vi "add delta initalize(SubVI).vi"(9 "字符串":string, 10 "model":string="Delta") -> (0 "连接的字符串":string, 3 "ok or cancel":bool=TRUE)   [LabVIEW 2019, in "Add Seq.lvlib"]
uses:
  Add Seq.lvlib
  lib/Keithley 622x/Configure/Delta PDelta DCon Modes/Typedefs/KE622x -- Delta Mode Params.ctl
  lib/Keithley 622x/Configure/Delta PDelta DCon Modes/Low Level/Typedefs/KE622x -- Delta PDelta Mode High Level.ctl
  lib/Keithley 622x/Configure/Delta PDelta DCon Modes/Low Level/Typedefs/KE622x -- Delta PDelta Mode Low Level.ctl
  lib/Keithley 622x/Configure/Delta PDelta DCon Modes/Low Level/Typedefs/KE622x -- Delta DCon Mode Delay.ctl
  lib/Keithley 622x/Configure/Delta PDelta DCon Modes/Low Level/Typedefs/KE622x -- Delta PDelta Mode Num Cycles Mode.ctl
  lib/Keithley 622x/Configure/Delta PDelta DCon Modes/Low Level/Typedefs/KE622x -- Delta PDelta Mode Num Cycles.ctl
  lib/Keithley 622x/Configure/2182 -A/Low Level/Typedefs/KE2182 -- Voltage Ranges.ctl
  lib/Keithley 622x/Configure/2182 -A/Low Level/Typedefs/KE2182 -- Filter Type.ctl
  lib/Keithley 622x/Configure/2182 -A/Low Level/Typedefs/KE2182 -- Filter Count.ctl
  lib/Keithley 622x/Configure/2182 -A/Low Level/Typedefs/KE2182 -- Filter Window.ctl
  lib/Keithley 622x/Configure/2182 -A/Low Level/Typedefs/KE2182 -- NPLCs.ctl
  SubVI.lvlib
  lib/Keithley 622x/Keithley 622x.lvlib
panel:
  out "错误输出":errorcluster
  in  "load":bool
  in  "2812 -A Params In":T6={"Auto Range?"=FALSE, "Man / Selected\nRange"=enum."10mV", "Enable Digital\nFilter?"=FALSE, "Filter Type"=enum."Moving", "Filter Count"=10, "Filter\nWindow (%)"=0.01, "Enable Analog\nFilter?"=FALSE, "NPLCs"=5} {"Filter\nWindow (%)" min=0.0 max=10.0 step=0.01 format="%.2f"; "Filter Count" min=1 max=100; "NPLCs" min=1 max=10}
  in  "Delta Mode Params In":T7={"High Level (A)"=0.001, "Low Level (A)"=-0.001, "Delay (s)"=0.02, "Num Cycles Mode"=enum."Finite Count", "Finite Count"=6, "Abort On\nCompliance?"=FALSE, "Cold Swithing\nMode Enabled?"=FALSE} {"Finite Count" min=1 max=65536; "Low Level (A)" min=-0.105 max=0.0 format="%.3p"; "High Level (A)" min=0.0 max=0.105 format="%.3p"; "Delay (s)" min=0.001 max=9999.999 format="%.3f"}
  in  "cancel":bool
  in  "ok":bool
  in  "6221 Resource":refnum<visa-resource-name>="GPIB1::10::INSTR"
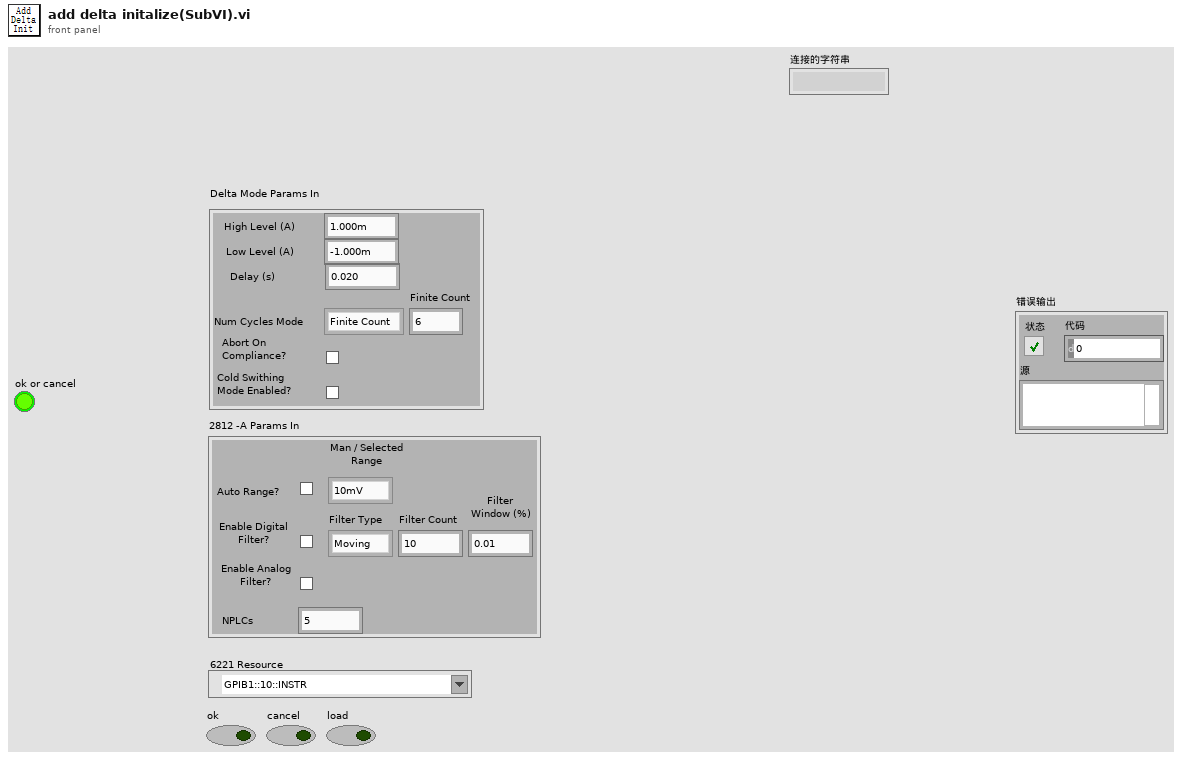
[diagram p1: front panel]
types:
  T1 = typedef "Keithley 622x.lvlib/KE2182 -- Voltage Ranges.ctl" = enum16{"10mV", "100mV", "1V", "10V", "100V"}
  T2 = typedef "Keithley 622x.lvlib/KE2182 -- Filter Type.ctl" = enum16{"Moving", "Repeat"}
  T3 = typedef "Keithley 622x.lvlib/KE2182 -- Filter Count.ctl" = u32
  T4 = typedef "Keithley 622x.lvlib/KE2182 -- Filter Window.ctl" = dbl
  T5 = typedef "Keithley 622x.lvlib/KE2182 -- NPLCs.ctl" = u32
  T6 = cluster{"Auto Range?":bool, "Man / Selected\nRange":T1, "Enable Digital\nFilter?":bool, "Filter Type":T2, "Filter Count":T3, "Filter\nWindow (%)":T4, "Enable Analog\nFilter?":bool, "NPLCs":T5}
  T7 = typedef "Keithley 622x.lvlib/KE622x -- Delta Mode Params.ctl" = cluster{"High Level (A)":T8, "Low Level (A)":T9, "Delay (s)":T10, "Num Cycles Mode":T11, "Finite Count":T12, "Abort On\nCompliance?":bool, "Cold Swithing\nMode Enabled?":bool}
  T8 = typedef "Keithley 622x.lvlib/KE622x -- Delta PDelta Mode High Level.ctl" = dbl
  T9 = typedef "Keithley 622x.lvlib/KE622x -- Delta PDelta Mode Low Level.ctl" = dbl
  T10 = typedef "Keithley 622x.lvlib/KE622x -- Delta DCon Mode Delay.ctl" = dbl
  T11 = typedef "Keithley 622x.lvlib/KE622x -- Delta PDelta Mode Num Cycles Mode.ctl" = enum16{"Finite Count", "Infinite"}
  T12 = typedef "Keithley 622x.lvlib/KE622x -- Delta PDelta Mode Num Cycles.ctl" = u32
  T13 = enum16{"open", "replace", "create", "open or create", "replace or create"}
  T14 = enum16{"open", "replace", "create", "open or create", "replace or create", "replace or create with confirmation"}
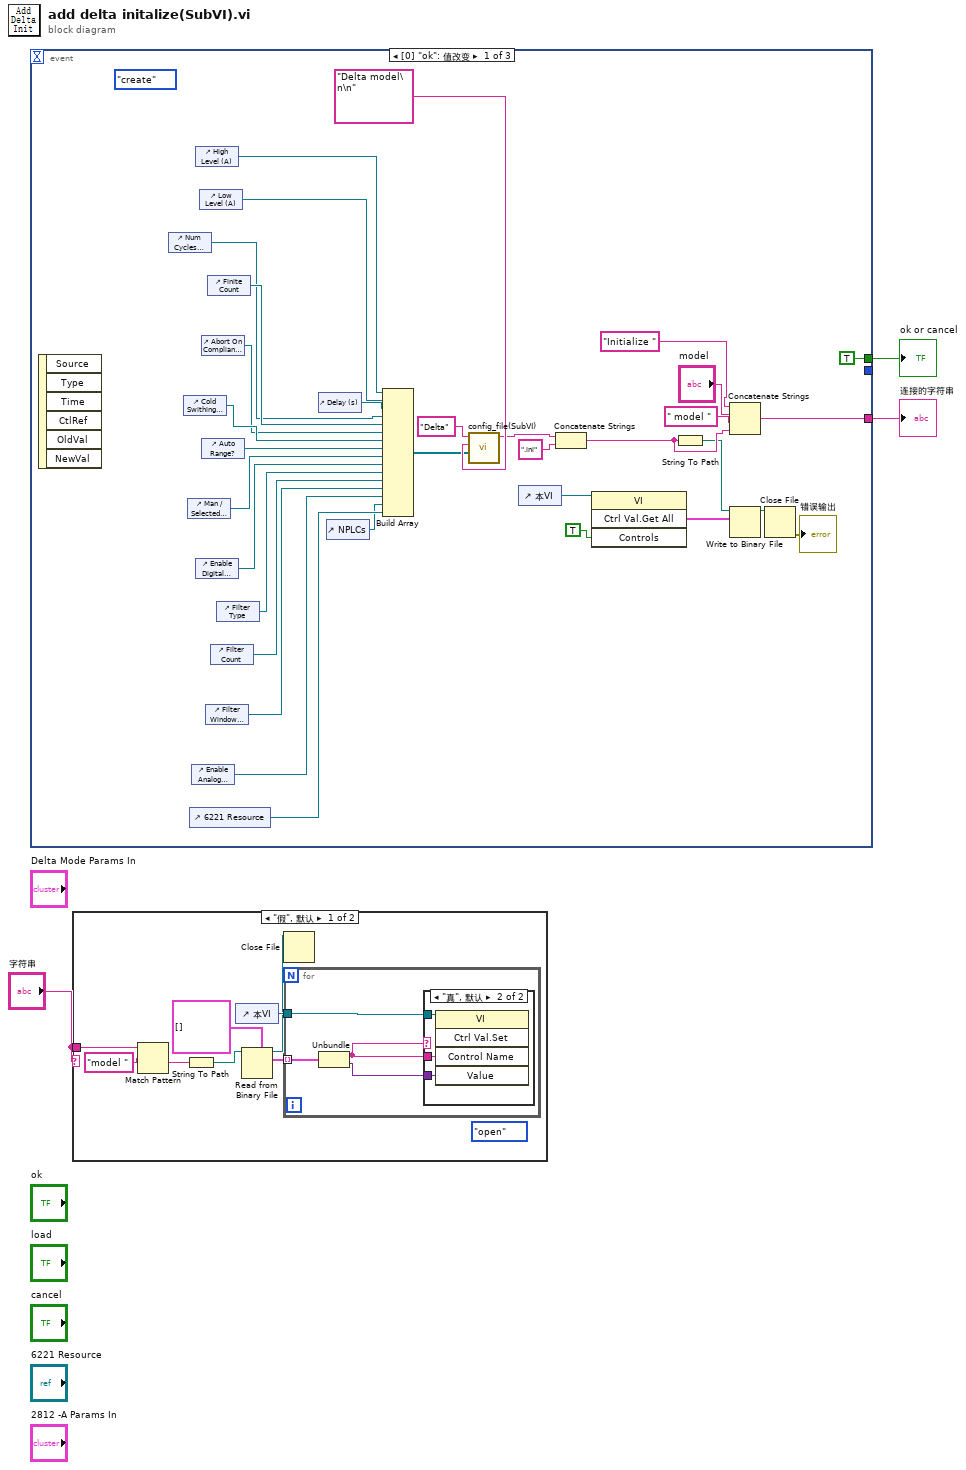
[diagram p0: block diagram]
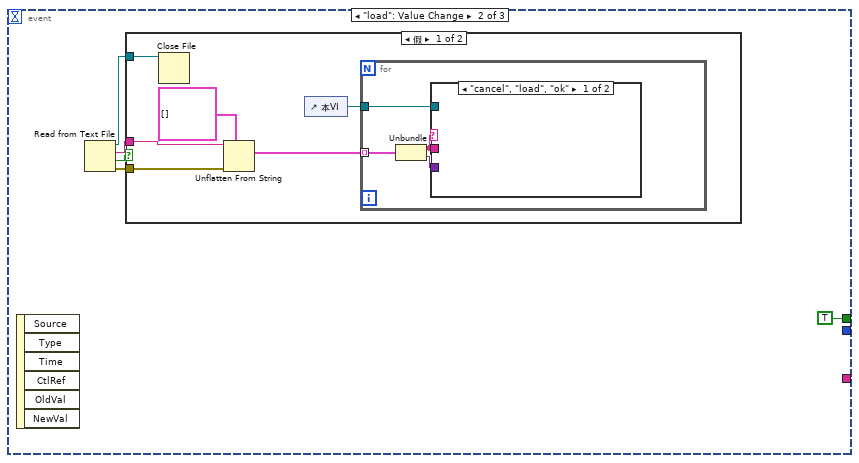
[diagram p4: hidden frame]
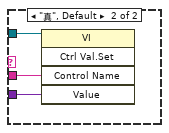
[diagram p5: hidden frame]
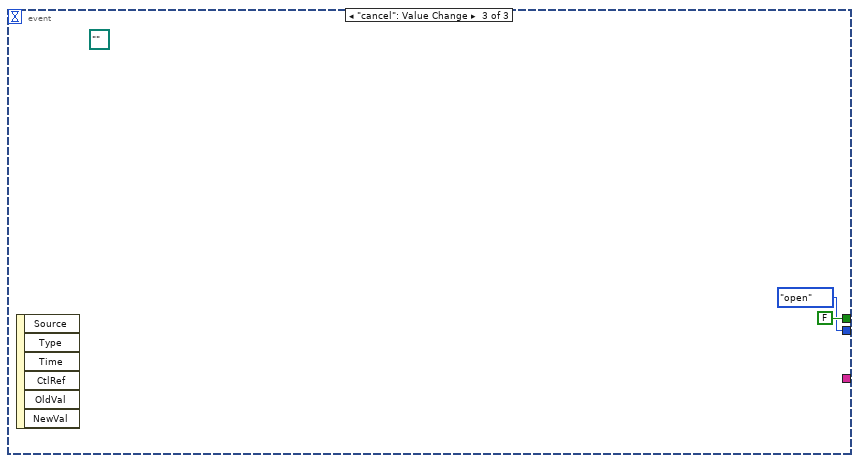
[diagram p7: hidden frame]
diagram:
  n1 = event shown="[0] \"ok\": 值改变" {
    selector: _ -> [_ _ _]
    dyn-events: _ -> [_ _ _]
    timeout: _ -> [_ _ _]
    tunnel: [_ _ T13."open" ("operation(0:open)")] -> _
    tunnel: [TRUE TRUE FALSE] -> w3
    tunnel: [w7 _ _] -> w2
    event "ok": Value Change {
      (unwired) T14."create" ("操作(0:open)")
      n2 = event-data() -> ()  [unwired: 1 in, 6 out]
      n3 = control-ref of="Num Cycles Mode"() -> (w15:refnum<vi>)
      n4 = control-ref of="Cold Swithing\nMode Enabled?"() -> (w18:refnum<vi>)
      n5 = control-ref of="Man / Selected\nRange"() -> (w20:refnum<vi>)
      n6 = control-ref of="6221 Resource"() -> (w27:refnum<vi>)
      n7 = control-ref of="Enable Analog\nFilter?"() -> (w25:refnum<vi>)
      n8 = control-ref of="High Level (A)"() -> (w12:refnum<vi>)
      n9 = control-ref of="Enable Digital\nFilter?"() -> (w21:refnum<vi>)
      n10 = control-ref of="Low Level (A)"() -> (w13:refnum<vi>)
      n11 = control-ref of="Abort On\nCompliance?"() -> (w17:refnum<vi>)
      n12 = control-ref of="Auto Range?"() -> (w19:refnum<vi>)
      n13 = control-ref of="Filter\nWindow (%)"() -> (w24:refnum<vi>)
      n14 = control-ref of="Finite Count"() -> (w16:refnum<vi>)
      n15 = control-ref of="Filter Count"() -> (w23:refnum<vi>)
      n16 = control-ref of="Filter Type"() -> (w22:refnum<vi>)
      n17 = control-ref of="Delay (s)"() -> (w14:refnum<vi>)
      n18 = control-ref of="NPLCs"() -> (w26:refnum<vi>)
      n19 = Build Array(w12, w13, w14, w15, w16, w17, w18, w19, w20, w21, w22, w23, w24, w25, w26, w27) -> (w10:refnum<vi>[])
      n20 = call "config_file(SubVI).vi"("all ref"=w10, "文件抬头"="Delta model\n\n", "文件夹名称"="Delta" ("字符串")) -> ("字符串输出"=w30:string)  [unwired: 8 in]
      n21 = control-ref of="本VI"() -> (w33:refnum<vi>)
      n22 = Concatenate Strings(w30, ".ini" ("字符串")) -> (w28:string)
      n23 = invoke class="VI" method="Ctrl Val.Get All"(reference=w33, "Controls"=TRUE ("控件")) -> ("Get All Control Values Variant"=w5:cluster{"Name":string, "Variant Data":variant}[])  [unwired: 2 in, 3 out]
      n24 = String To Path(string=w28) -> (path=w6:path)
      n25 = Concatenate Strings("Initialize " ("字符串"), "model", " model " ("字符串"), w28) -> (w7:string)
      n26 = Write to Binary File(file (use dialog)=w6, data=w5) -> (refnum out=w4:refnum<file>)  [unwired: 4 in, 2 out]
      n27 = Close File(refnum=w4) -> (error out=→"错误输出":errorcluster)  [unwired: 1 in, 1 out]
    }
    event "load": Value Change {
      n28 = event-data() -> ()  [unwired: 1 in, 6 out]
      n29 = Read from Text File() -> (refnum out=w40:refnum<file>, text=w38:string, cancelled=w37:bool, error out=w39:errorcluster)  [unwired: 4 in]
      n30 = case shown="假" w37 {
        tunnel: w40 -> [w47 _]
        tunnel: w39 -> [w45 _]
        tunnel: w38 -> [w44 _]
        frame False {
          n31 = Close File(refnum=w47) -> ()  [unwired: 1 in, 2 out]
          n32 = Unflatten From String(type=cluster{"Name":string, "Variant Data":variant}[] [] ("控件值:获取全部"), binary string=w44, error in (no error)=w45) -> (value=w43:cluster{"Name":string, "Variant Data":variant}[])  [unwired: 2 in, 2 out]
          n33 = control-ref of="本VI"() -> (w42:refnum<vi>)
          n34 = for {
            tunnel: w43 -> [w51] mode=indexing
            tunnel: w42 -> [w50]
            n35 = Unbundle(w51) -> ("Name"=w48:string, "Variant Data"=w49:variant)
            n36 = case shown="\"cancel\", \"load\", \"ok\"" w48 {
              tunnel: w50 -> [_ w54]
              tunnel: w48 -> [_ w53]
              tunnel: w49 -> [_ w52]
              frame "cancel", "load", "ok" {
              }
              frame "真", Default {
                n37 = invoke class="VI" method="Ctrl Val.Set"(reference=w54, "Control Name"=w53, "Value"=w52) -> ()  [unwired: 2 in, 5 out]
              }
            }
          }
        }
        frame True {
        }
      }
    }
    event "cancel": Value Change {
      (unwired) path "" ("path")
      n38 = event-data() -> ()  [unwired: 1 in, 6 out]
    }
  }
  "ok or cancel" <- w3
  "连接的字符串" <- w2
  n39 = case shown="\"假\", 默认" "字符串" {
    tunnel: "字符串" -> [w64 _]
    frame "假", Default {
      (unwired) T14."open" ("操作(0:open)")
      n40 = Match Pattern(string=w64, regular expression="model " ("正则表达式")) -> (after substring=w63:string)  [unwired: 1 in, 3 out]
      n41 = String To Path(string=w63) -> (path=w60:path)
      n42 = control-ref of="本VI"() -> (w61:refnum<vi>)
      n43 = Read from Binary File(5:cluster{"Name":string, "Variant Data":variant}[] [] ("控件值:获取全部"), 11:w60) -> (2:w58:cluster{"Name":string, "Variant Data":variant}[], 3:w57:refnum<file>)  [unwired: 4 in, 2 out]
      n44 = Close File(refnum=w57) -> ()  [unwired: 1 in, 2 out]
      n45 = for {
        tunnel: w58 -> [w68] mode=indexing
        tunnel: w61 -> [w67]
        n46 = Unbundle(w68) -> ("Name"=w65:string, "Variant Data"=w66:variant)
        n47 = case shown="\"真\", 默认" w65 {
          tunnel: w67 -> [_ w71]
          tunnel: w65 -> [_ w70]
          tunnel: w66 -> [_ w69]
          frame "cancel", "load", "ok" {
          }
          frame "真", Default {
            n48 = invoke class="VI" method="Ctrl Val.Set"(reference=w71, "Control Name"=w70, "Value"=w69) -> ()  [unwired: 2 in, 5 out]
          }
        }
      }
    }
    frame "" {
    }
  }
